vi "Sound Files.vi"() -> ()   [LabVIEW 2009]
panel:
  out "temperaturelimit":path=path "C:/LabVIEW John/Sound/XP Sounds/tada.wav"
  out "xpexcl":path=path "C:/LabVIEW/Sound/XP Sounds/Windows XP Exclamation.wav"
  out "xpnotify":path=path "C:/LabVIEW/Sound/XP Sounds/Windows XP Notify.wav"
  out "xperror":path=path "C:/LabVIEW/Sound/XP Sounds/Windows XP Error.wav"
  out "xpding":path=path "C:/LabVIEW/Sound/XP Sounds/Windows XP Ding.wav"
  out "critstop":path=path "C:/LabVIEW/Sound/XP Sounds/Windows XP Critical Stop.wav"
  out "battlow":path=path "C:/LabVIEW/Sound/XP Sounds/Windows XP Battery Low.wav"
  out "battcrit":path=path "C:/LabVIEW/Sound/XP Sounds/Windows XP Battery Critical.wav"
  out "tada":path=path "C:/LabVIEW/Sound/XP Sounds/tada.wav"
  out "notify":path=path "C:/LabVIEW/Sound/XP Sounds/notify.wav"
  out "chord":path=path "C:/LabVIEW/Sound/XP Sounds/Chord.wav"
  out "ding":path=path "C:/LabVIEW/Sound/XP Sounds/ding.wav"
  out "startup":path=path "C:/LabVIEW/Sound/Voice/startup.wav"
  out "goodbye":path=path "C:/LabVIEW/Sound/Voice/goodbye.wav"
  out "train":path=path "C:/LabVIEW/Sound/Voice/train.wav"
  out "terminated":path=path "C:/LabVIEW/Sound/Voice/terminated.wav"
  out "notready":path=path "C:/LabVIEW/Sound/Voice/scan not ready.wav"
  out "scanint":path=path "C:/LabVIEW/Sound/Voice/scan interrupt.wav"
  out "scancancel":path=path "C:/LabVIEW/Sound/Voice/scan cancel.wav"
  out "error":path=path "C:/LabVIEW/Sound/Voice/error.wav"
  out "scanbelong":path=path "C:/LabVIEW/Sound/Voice/scan belong.wav"
  out "PClimit":path=path "C:/LabVIEW/Sound/Voice/PC limit.wav"
  out "pause":path=path "C:/LabVIEW/Sound/Voice/pause.wav"
  out "lowcryo":path=path "C:/LabVIEW/Sound/Voice/low cryogens.wav"
  out "danger":path=path "C:/LabVIEW/Sound/Voice/danger.wav"
  out "allscans":path=path "C:/LabVIEW/Sound/Voice/all scans done.wav"
  out "scandone":path=path "C:/LabVIEW/Sound/Voice/scan done.wav"
  out "sweepint":path=path "C:/LabVIEW/Sound/Voice/sweep interrupt.wav"
  out "leavepersis":path=path "C:/LabVIEW/Sound/Voice/leave persistent.wav"
  out "enterpersis":path=path "C:/LabVIEW/Sound/Voice/enter persistent.wav"
  out "zero":path=path "C:/LabVIEW/Sound/Voice/at zero.wav"
  out "field":path=path "C:/LabVIEW/Sound/Voice/at field.wav"
  out "lvlN":path=path "C:/LabVIEW/Sound/Voice/N lvl hit.wav"
  out "lvlHe":path=path "C:/LabVIEW/Sound/Voice/He lvl hit.wav"
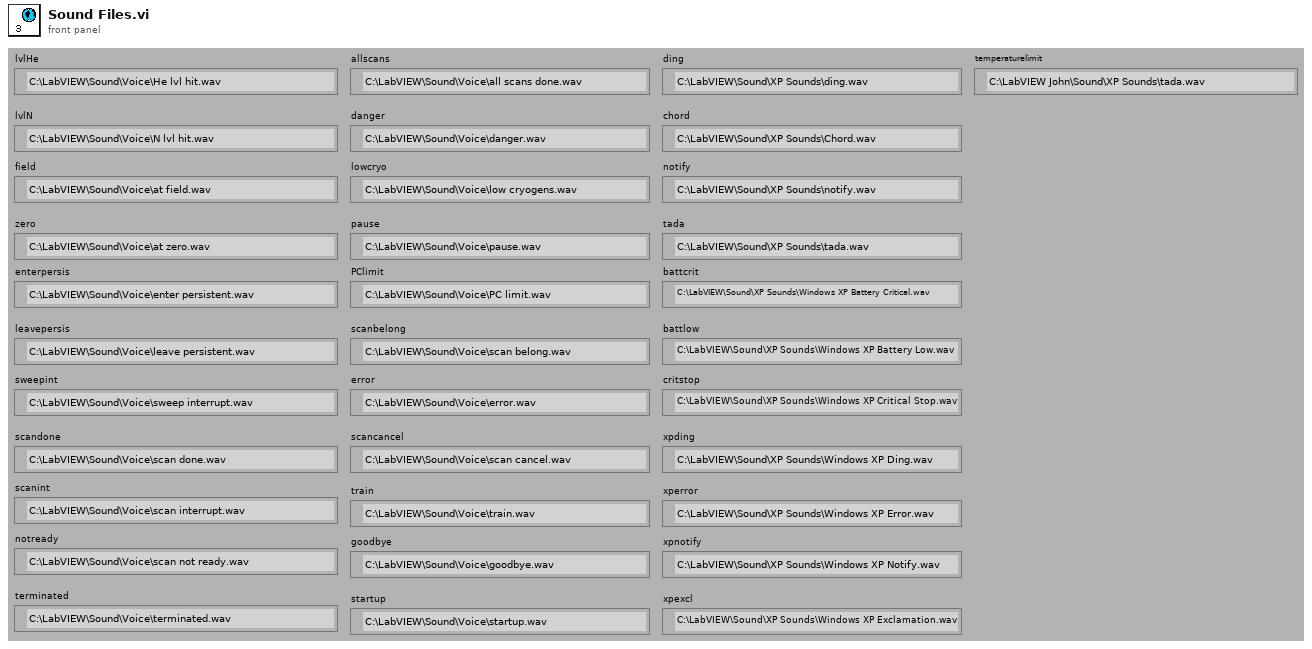
[diagram p1: front panel]
diagram:
